vi "get Class Data.vi"(8 "Error In":errorcluster, 10 "Selected Instance":string, 11 "Instance Data Array":T1[](array[typedef])) -> (0 "Error Out":errorcluster)   [LabVIEW 2019, in "Arithemetic Operation.lvclass"]
doc: "This method gets the data of the instance searched by the user."
uses:
  Arithemetic Operation.lvclass
  Typedef/User Event Operations.ctl
  Typedef/Class Data.ctl
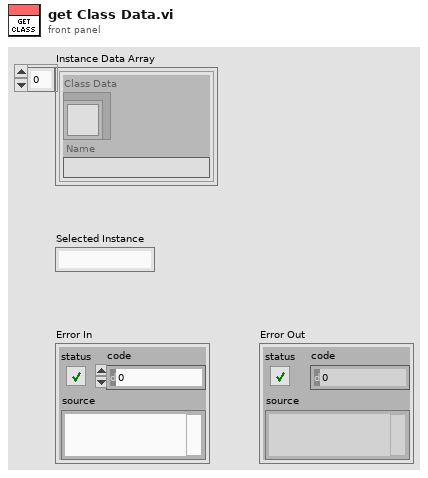
[diagram p1: front panel]
types:
  T1 = typedef "Class Data.ctl" = cluster{"Class Data":refnum<class "Arithemetic Operation.lvclass">, "Name":string}
  T2 = typedef "User Event Operations.ctl" = enum16{"Obtain", "Generate", "Destroy"}
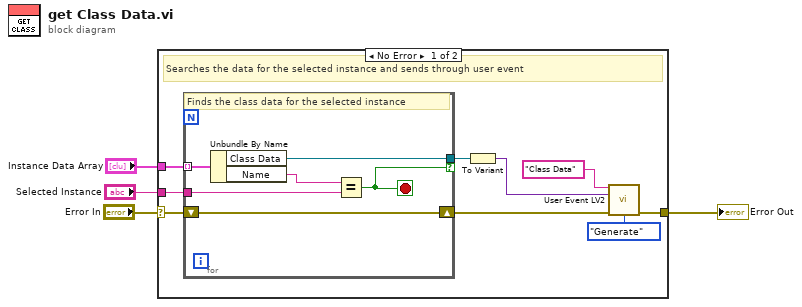
[diagram p0: block diagram]
diagram:
  n1 = case shown="No Error" "Error In" {
    selector: "Error In" -> [w10 w20]
    tunnel: [w11 w20] -> w3
    tunnel: "Instance Data Array" -> [w9 _]
    tunnel: "Selected Instance" -> [w8 _]
    frame No Error {
      # "Searches the data for the selected instance and sends through user event"
      n2 = for {
        tunnel: w9 -> [w19] mode=indexing
        tunnel: [w17] -> w7 if=w15
        tunnel: w8 -> [w14]
        shift-right: [w16] -> w13
        shift-left: w10 -> [w16]
        stop <- w15 stop-if-true
        # "Finds the class data for the selected instance"
        n3 = Unbundle By Name(w19) -> ("Class Data"=w17:refnum<class "Arithemetic Operation.lvclass">, "Name"=w18:string)
        n4 = Equal?(x=w18, y=w14) -> (x = y?=w15:bool)
      }
      n5 = To Variant(anything=w7) -> (Variant=w6:variant)
      n6 = call "User Event LV2.vi"("Event Name"="Class Data", "Data"=w6, "Error In"=w13, "Operation"=User_Event_Operations."Generate") -> ("Error Out"=w11:errorcluster)  [unwired: 10 in, 1 out]
    }
    frame Error {
    }
  }
  "Error Out" <- w3
